vi "mod_Arrange QAM Symbols.vi"(1 "columns":u32, 2 "rows":u32, 3 "Gray coded values":i32[](array[numeric])) -> (0 "Symbol Values":i32[][](array[numeric]))   [LabVIEW 2020, in "niDMT.lvlib"]
uses:
  <vilib>/addons/Modulation/niDMT.lvlib
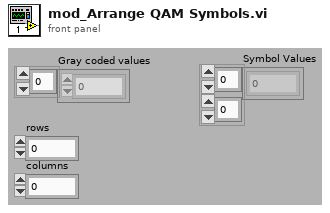
[diagram p1: front panel]
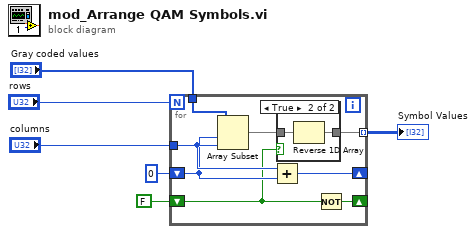
[diagram p0: block diagram]
diagram:
  n1 = for {
    N: "rows" -> [_]
    tunnel: "Gray coded values" -> [w14]
    shift-right: [w8] -> _
    shift-left: FALSE -> [w7]
    tunnel: "columns" -> [w12]
    shift-right: [w13] -> _
    shift-left: 0 -> [w11]
    tunnel: [w9] -> w6 mode=indexing
    n2 = Array Subset(array=w14, index=w11, length=w12) -> (w10:i32[])
    n3 = Add(x=w12, y=w11) -> (x+y=w13:u32)
    n4 = case shown="True" w7 {
      tunnel: w10 -> [w15 w17]
      tunnel: [w15 w16] -> w9
      frame False {
      }
      frame True {
        n5 = Reverse 1D Array(array=w17) -> (reversed array=w16:i32[])
      }
    }
    n6 = Not(x=w7) -> (.not. x?=w8:bool)
  }
  "Symbol Values" <- w6
